vi "kinectRead [Infrared Frame].vi"(8 "error in (no error)":errorcluster, 9 "Timeout (ms)":i32=5000, 11 "KinectSensor References in":T1) -> (0 "error out":errorcluster, 2 "frameData":u16[](array[numeric]), 3 "KinectSensor References out":T1)   [LabVIEW 2014]
uses:
  controls/KinectSensor References.ctl
  Microsoft.Kinect
  C:/github/labviewhacker/LVH-KinectOne/LabVIEW/vi.lib/LabVIEW Hacker/KinectOne/support/BodyFrameDataInterface.dll
  BodyFrameDataInterface.dll
  Frame Data FGV [Infrared].vi
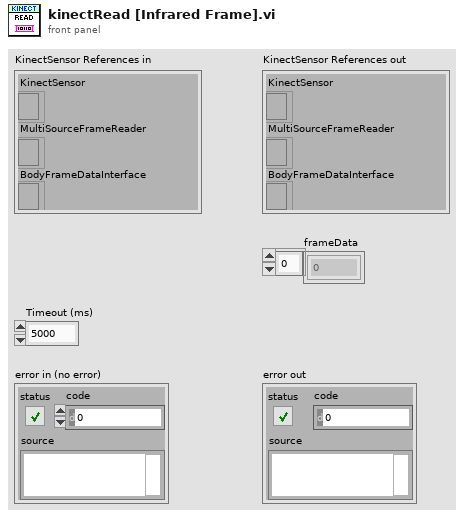
[diagram p1: front panel]
types:
  T1 = typedef "KinectSensor References.ctl" = cluster{"KinectSensor":refnum<k24>, "MultiSourceFrameReader":refnum<k24>, "BodyFrameDataInterface":refnum<k24>}
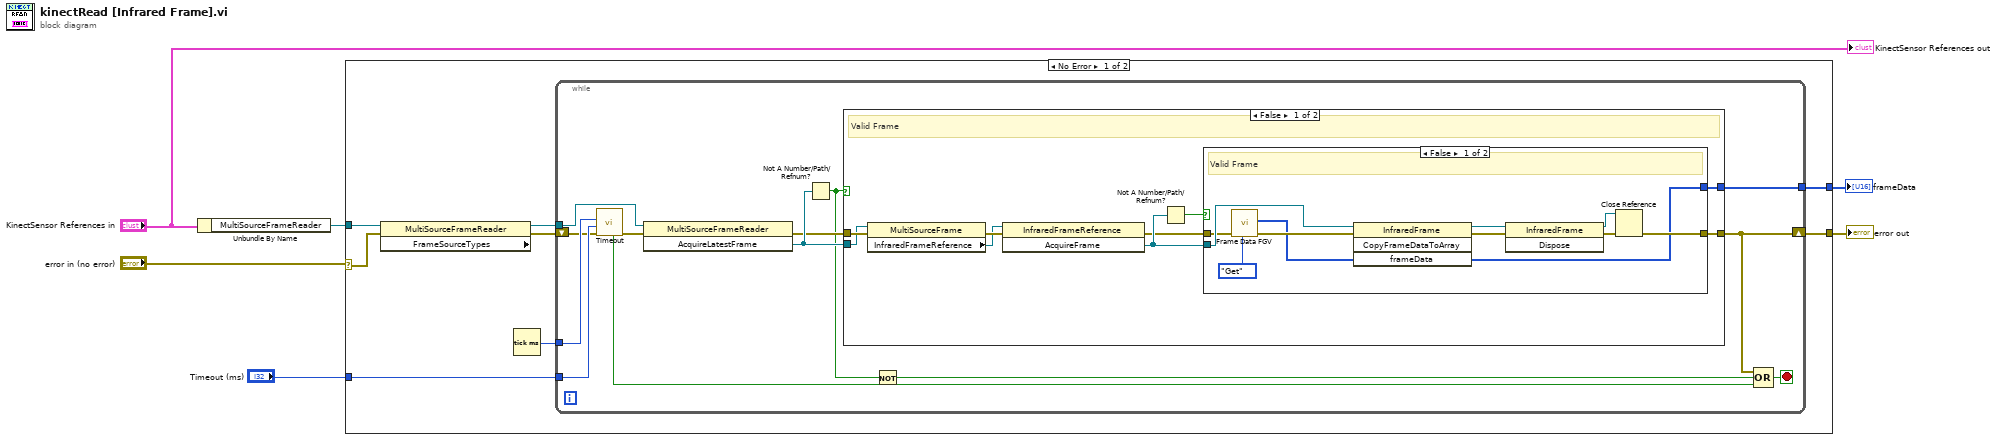
[diagram p0: block diagram]
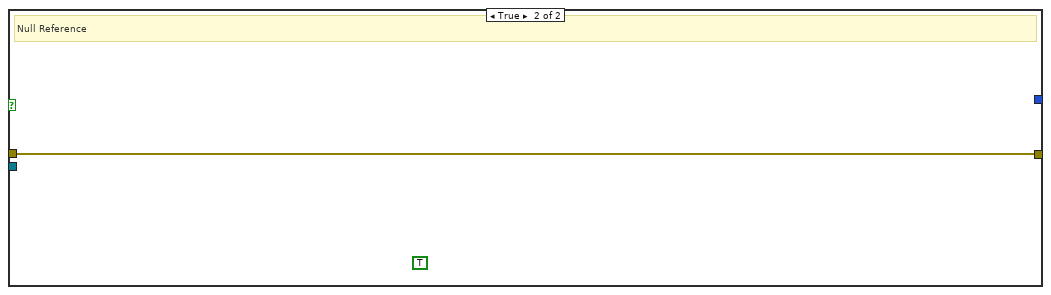
[diagram p3: hidden frame]
diagram:
  n1 = Unbundle By Name("KinectSensor References in") -> ("MultiSourceFrameReader"=w6:refnum<k24>)
  n2 = case shown="No Error" "error in (no error)" {
    selector: "error in (no error)" -> [w9 w50]
    tunnel: w6 -> [w12 _]
    tunnel: [w11 w50] -> w1
    tunnel: [w10 _] -> w4
    tunnel: "Timeout (ms)" -> [w7 _]
    frame No Error {
      n3 = property class="MultiSourceFrameReader" props=["FrameSourceTypes"](reference=w12, error in=w9) -> (reference out=w14:refnum<k24>, error out=w13:errorcluster)  [unwired: 1 out]
      n4 = Tick Count (ms)() -> (millisecond timer value=w8:u32)
      n5 = while {
        tunnel: w14 -> [w20]
        shift-right: [w18] -> w11
        shift-left: w13 -> [w22]
        tunnel: [w25] -> w10
        tunnel: w8 -> [w24]
        tunnel: w7 -> [w23]
        stop <- w17 stop-if-true
        n6 = call "Timeout.vi"("error in (no error)"=w22, "Timeout (ms)"=w23, "Start Time"=w24) -> ("error out"=w21:errorcluster, "Timeout?"=w19:bool)  [unwired: 7 in]
        n7 = invoke class="MultiSourceFrameReader" method="AcquireLatestFrame"(reference=w20, error in=w21) -> (error out=w26:errorcluster, "AcquireLatestFrame"=w27:refnum<k24>)  [unwired: 1 in, 1 out]
        n8 = Not A Number/Path/Refnum?(number/path/refnum=w27) -> (NaN/Path/Refnum?=w16:bool)
        n9 = case shown="False" w16 {
          tunnel: w26 -> [w33 w49]
          tunnel: w27 -> [w30 _]
          tunnel: [w32 w49] -> w18
          tunnel: [w28 _] -> w25
          frame False {
            # "Valid Frame"
            n10 = property class="MultiSourceFrame"(reference=w30, error in=w33) -> (error out=w34:errorcluster, "InfraredFrameReference"=w29:refnum<k24>)  [unwired: 1 out]
            n11 = invoke class="InfraredFrameReference" method="AcquireFrame"(reference=w29, error in=w34) -> (error out=w35:errorcluster, "AcquireFrame"=w36:refnum<k24>)  [unwired: 1 in, 1 out]
            n12 = Not A Number/Path/Refnum?(number/path/refnum=w36) -> (NaN/Path/Refnum?=w31:bool)
            n13 = case shown="False" w31 {
              tunnel: w35 -> [w40 w48]
              tunnel: w36 -> [w43 _]
              tunnel: [w42 w48] -> w32
              tunnel: [w41 _] -> w28
              frame False {
                # "Valid Frame"
                n14 = call-poly "Frame Data FGV.vi"("Command"=enum16{"Get", "Initialize"}."Get", "error in (no error)"=w40) -> ("error out"=w39:errorcluster, "Array"=w38:u16[])  [unwired: 8 in]
                n15 = invoke class="InfraredFrame" method="CopyFrameDataToArray"(reference=w43, error in=w39, "frameData"=w38) -> (reference out=w44:refnum<k24>, error out=w45:errorcluster, "frameData"=w41:u16[])  [unwired: 1 in, 1 out]
                n16 = invoke class="InfraredFrame" method="Dispose"(reference=w44, error in=w45) -> (reference out=w47:refnum<k24>, error out=w46:errorcluster)  [unwired: 1 in, 1 out]
                n17 = Close Reference(reference=w47, error in (no error)=w46) -> (error out=w42:errorcluster)
              }
              frame True {
                # "Null Reference"
              }
            }
          }
          frame True {
            (unwired) TRUE
            # "Null Reference"
          }
        }
        n18 = Not(x=w16) -> (.not. x?=w15:bool)
        n19 = Compound Arithmetic op=OR(w18, w15, w19) -> (w17:bool)
      }
    }
    frame Error {
      # "Pass out upstream error"
    }
  }
  "error out" <- w1
  "frameData" <- w4
  "KinectSensor References out" <- "KinectSensor References in"
